vi "Magic Tote Detect.vi"(10 "Image Dst Out":T1) -> ()   [LabVIEW 2014]
uses:
  <vilib>/vision/Image Controls.llb/IMAQ Image.ctl
  <vilib>/vision/NI_Vision_Development_Module.lvlib
panel:
  out "num matches":i32[](array[numeric])
  in  "Zone H":dbl=7.0 format="%#_13g"
  out "Image Out":T1
  out "Number of Matches":i32
  in  "Image Dst Out 2":T1
  out "Waveform Graph":T2(graph)
  out "Histogram Report 3":T3 {"Standard  Variation" format="%.2f"; "Mean Value" format="%.2f"; "Interval Width" format="%.2f"; "Starting Value" format="%.2f"; "Maximal Value" format="%.2f"; "Minimal Value" format="%.2f"}
  out "Blue or Luma or Val or Inten Plane out":T1(plugin-control)
  in  "Zone W":dbl=7.0 format="%#_13g"
  in  "Exam Zone Offset X":dbl
  in  "Exam Zone Offset Y":dbl
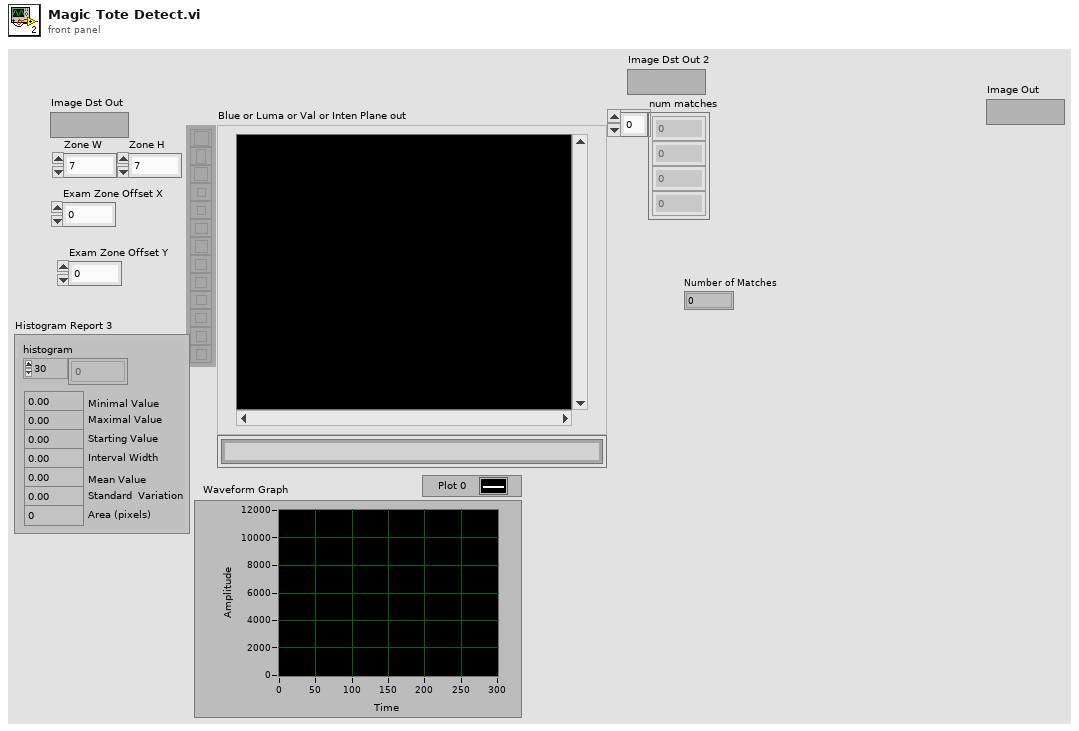
[diagram p1: front panel]
types:
  T1 = typedef "IMAQ Image.ctl" = refnum<image>
  T2 = cluster{"Starting Value":sgl, "Incremental Value":sgl, "Histogram":u32[]}
  T3 = cluster{"histogram":u32[], "Minimal Value":sgl, "Maximal Value":sgl, "Starting Value":sgl, "Interval Width":sgl, "Mean Value":sgl, "Standard  Variation":sgl, "Area (pixels)":i32}
  T4 = typedef "Image Type" = u32
  T5 = typedef "IMAQ Rectangle" = cluster{"Left":i32, "Top":i32, "Right":i32, "Bottom":i32, "Rotation":dbl}
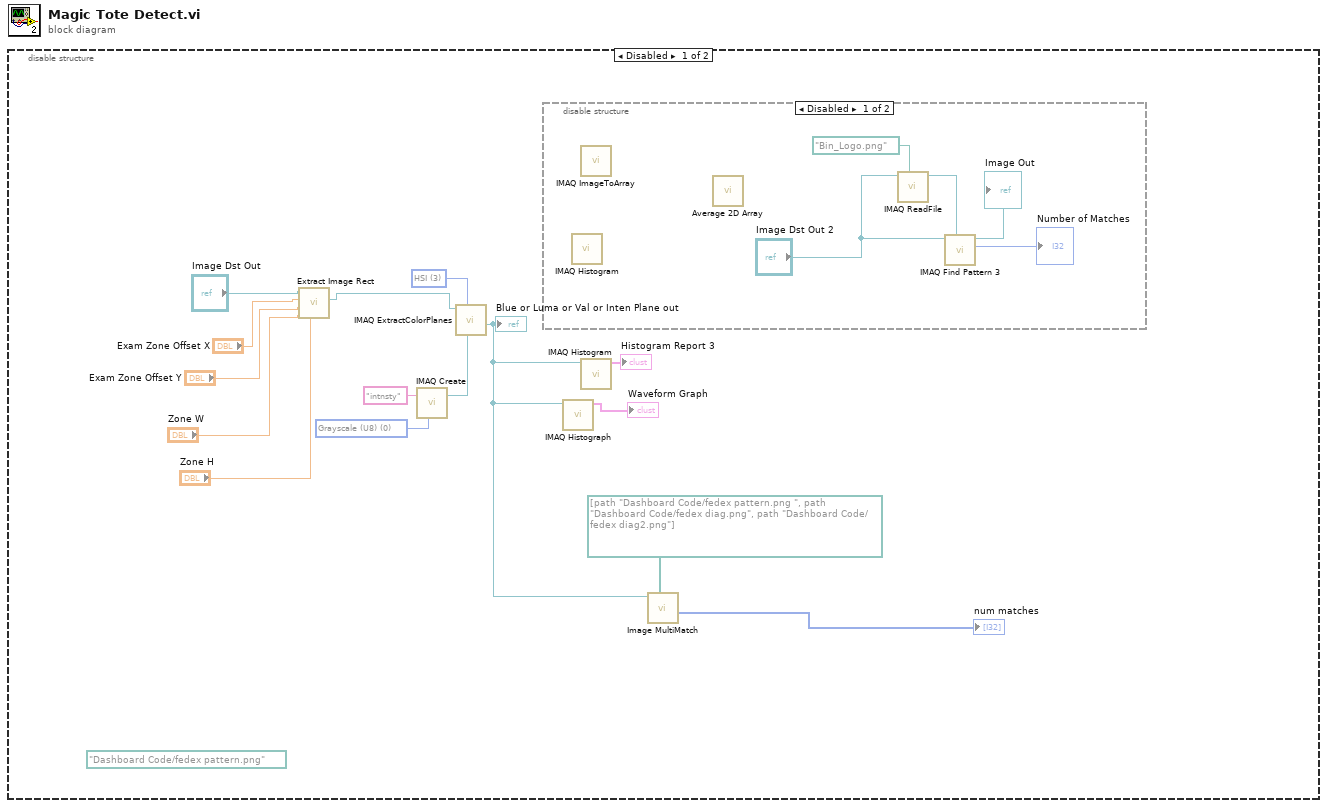
[diagram p0: block diagram]
diagram:
  n1 = disable-structure shown="Disabled" {
    frame Disabled {
      (unwired) path "Dashboard Code/fedex pattern.png" ("File Path")
      w13 = T4 0 items=["Grayscale (U8)", "Grayscale (I16)", "Grayscale (SGL)", "Complex (CSG)", "RGB (U32)", "HSL (U32)", "RGB (U64)", "Grayscale (U16)"] ("Image Type")
      w15 = u16 3 items=["RGB", "HSL", "HSV", "HSI"] ("Color Mode")
      n2 = call "Extract Image Rect.vi"("Zone H"="Zone H", "Zone W"="Zone W", "Exam Zone Offset Y"="Exam Zone Offset Y", "Exam Zone Offset X"="Exam Zone Offset X", "Source In"="Image Dst Out") -> ("Extracted Out"=w4:T1)  [unwired: 5 in, 1 out]
      n3 = call "IMAQ Create"("Image Name"="intnsty", "Image Type"=w13) -> ("New Image"=w12:T1)  [unwired: 3 in, 1 out]
      n4 = call "IMAQ ExtractColorPlanes"("Blue or Luma or Val or Inten Plane"=w12, "Color Mode"=w15, "Image Src"=w4) -> ("Blue or Luma or Val or Inten Plane out"=w2:T1)  [unwired: 5 in, 3 out]
      "Blue or Luma or Val or Inten Plane out" <- w2
      n5 = disable-structure shown="Disabled" {
        frame Disabled {
          n6 = call "IMAQ Histogram"() -> ()  [unwired: 10 in, 2 out]
          n7 = call "IMAQ ImageToArray"() -> ()  [unwired: 4 in, 5 out]
          n8 = call "Average 2D Array.vi"() -> ("Image Pixels (U8)"=w22:u8[][])  [unwired: 10 in, 1 out]
          n9 = call "IMAQ ReadFile"("File Path"=path "Bin_Logo.png", "Image"="Image Dst Out 2") -> ("Image Out"=w18:T1)  [unwired: 5 in, 4 out]
          n10 = call "IMAQ Find Pattern 3"("Template"=w18, "Image"="Image Dst Out 2") -> ("Number of Matches"=→"Number of Matches":i32, "Image Out"=→"Image Out":T1, "Search Rect"=w20:T5)  [unwired: 3 in, 4 out]
        }
        frame Enabled {
        }
      }
      n11 = call "IMAQ Histograph"("Image"=w2) -> ("Histogram Graph"=→"Waveform Graph":T2)  [unwired: 7 in, 3 out]
      n12 = call "IMAQ Histogram"("Image"=w2) -> ("Histogram Report"=→"Histogram Report 3":T3)  [unwired: 9 in, 1 out]
      n13 = call "Image MultiMatch.vi"("Image file paths"=path[] [path "Dashboard Code/fedex pattern.png ", path "Dashboard Code/fedex diag.png", path "Dashboard Code/fedex diag2.png"], "Refnum in"=w2) -> ("num matches"=→"num matches":i32[])  [unwired: 8 in, 1 out]
    }
    frame Enabled {
    }
  }
